vi "Raster Scan_2024-05-21+.vi"() -> ()   [LabVIEW 2024]
doc: "Shows how to move a motor to an absolute position."
uses:
  C:/Users/Behna/OneDrive/Desktop/Kinesis - Move Absolute- my work-with laser - Copy Folder/Thorlabs.MotionControl.Controls.dll
  Thorlabs.MotionControl.Controls.dll
  C:/Users/Behna/OneDrive/Desktop/Kinesis - Move Absolute- my work-with laser - Copy Folder/ThorLabs.MotionControl.KCube.DCServoCLI.dll
  ThorLabs.MotionControl.KCube.DCServoCLI.dll
  <vilib>/httpClient/LabVIEWHTTPClient.lvlib
panel:
  out "x .and. y?":bool
  in  "String":string
  out "Response":string
  in  "VISA resource name":refnum<visa-resource-name>="COM4"
  out "headers 2":string
  out "body 2":string
  out "laser run":i32
  out "remaining pulse":i32
  out "x*y":dbl
  out "GetMoveAbsolutePositionZ":dbl=6.0
  out "Numeric 2":i32
  out "Numeric":i32
  out "GetMoveAbsolutePositionX":dbl=6.0
  out "x = y?":bool
  in  "initial value_X":dbl=5.0
  in  "initial value_Z":dbl=4.0
  in  "Pulse number":string="200"
  out "body":string="{\"message\":\"success\"}"
  out "headers":string="HTTP/1.1 200 OK\r\nTransfer-Encoding: chunked\r\n\r\n"
  in  "Z-Step size":dbl=1.0
  in  "# Z-points":i32=2
  out "Z-Step":dbl[](array[numeric])=[1.0, 2.0, 3.0, 4.0, 5.0, 6.0]
  out "X-Step":dbl[](array[numeric])=[1.0, 2.0, 3.0, 4.0, 5.0, 6.0]
  in  "# X-points":i32=2
  in  "X-Step size":dbl=1.0
  in  "KCubeDCServoControl 2":refnum<k24>(container)
  in  "SerialNumber 2":string="27261646"
  in  "SerialNumber":string="27261828"
  in  "KCubeDCServoControl":refnum<k24>(container)
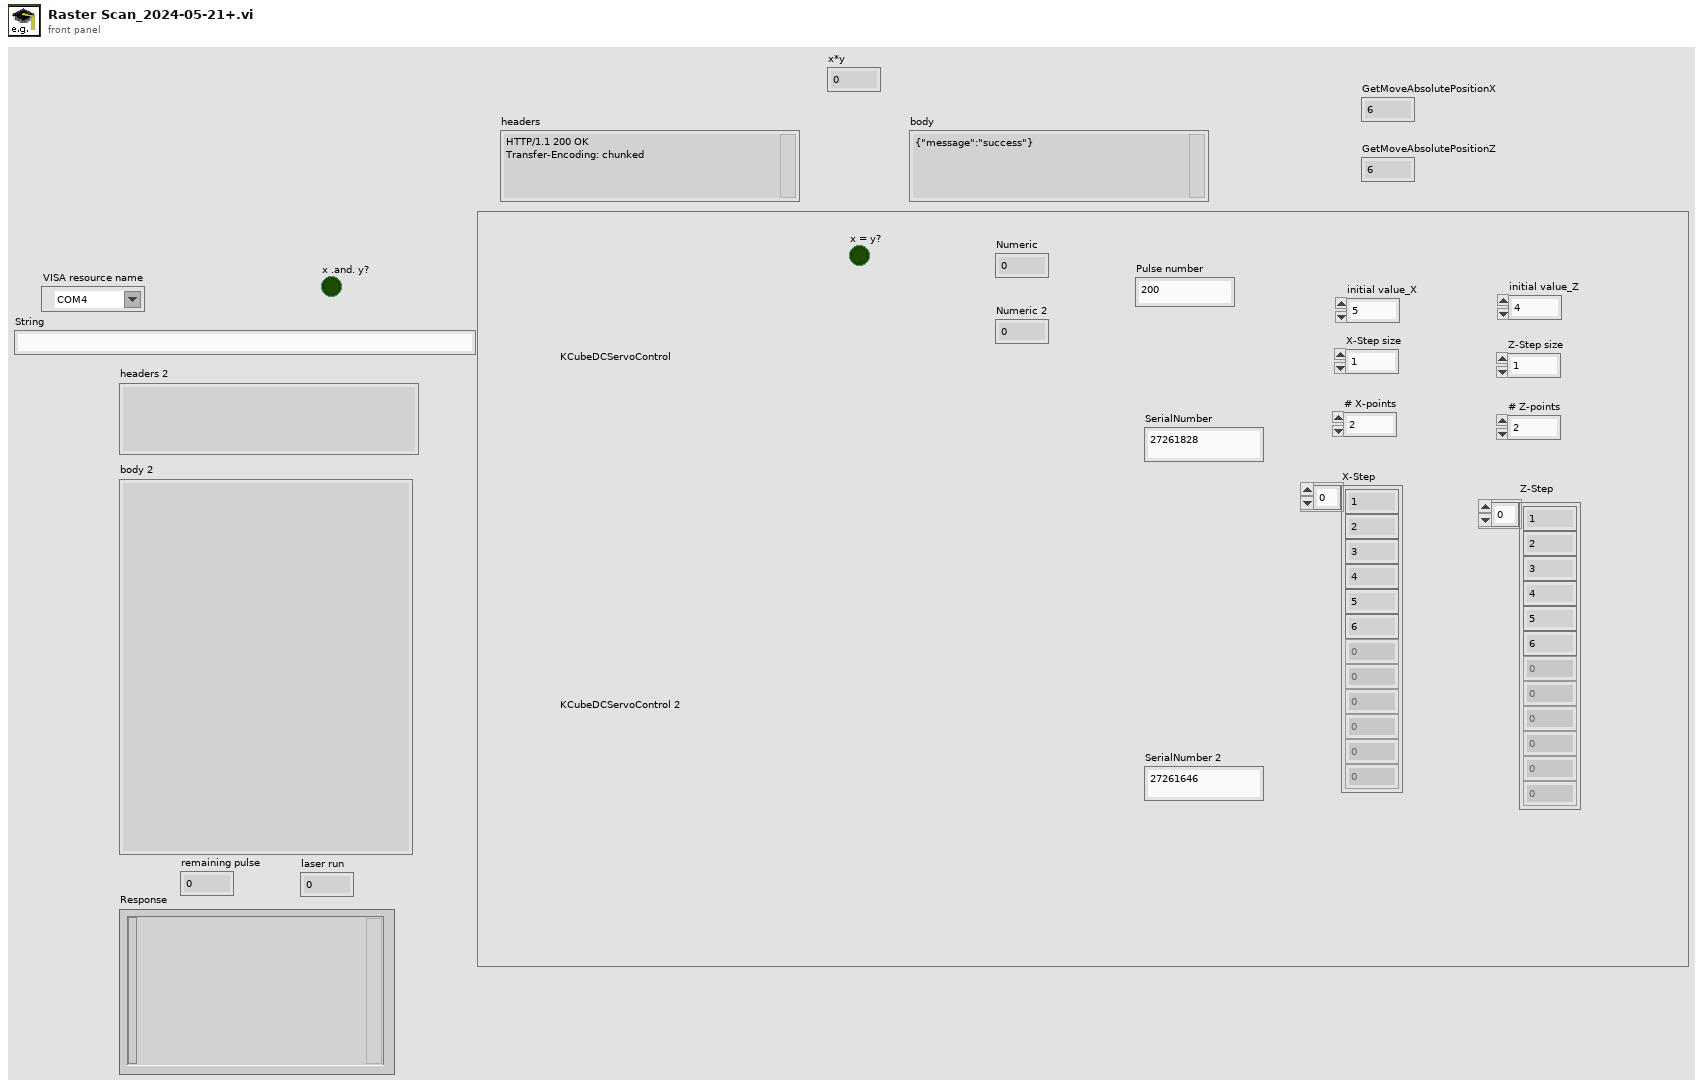
[diagram p1: front panel]
types:
  T1 = typedef "LabVIEWHTTPClient.lvlib/ClientHandle.ctl" = refnum<k1>
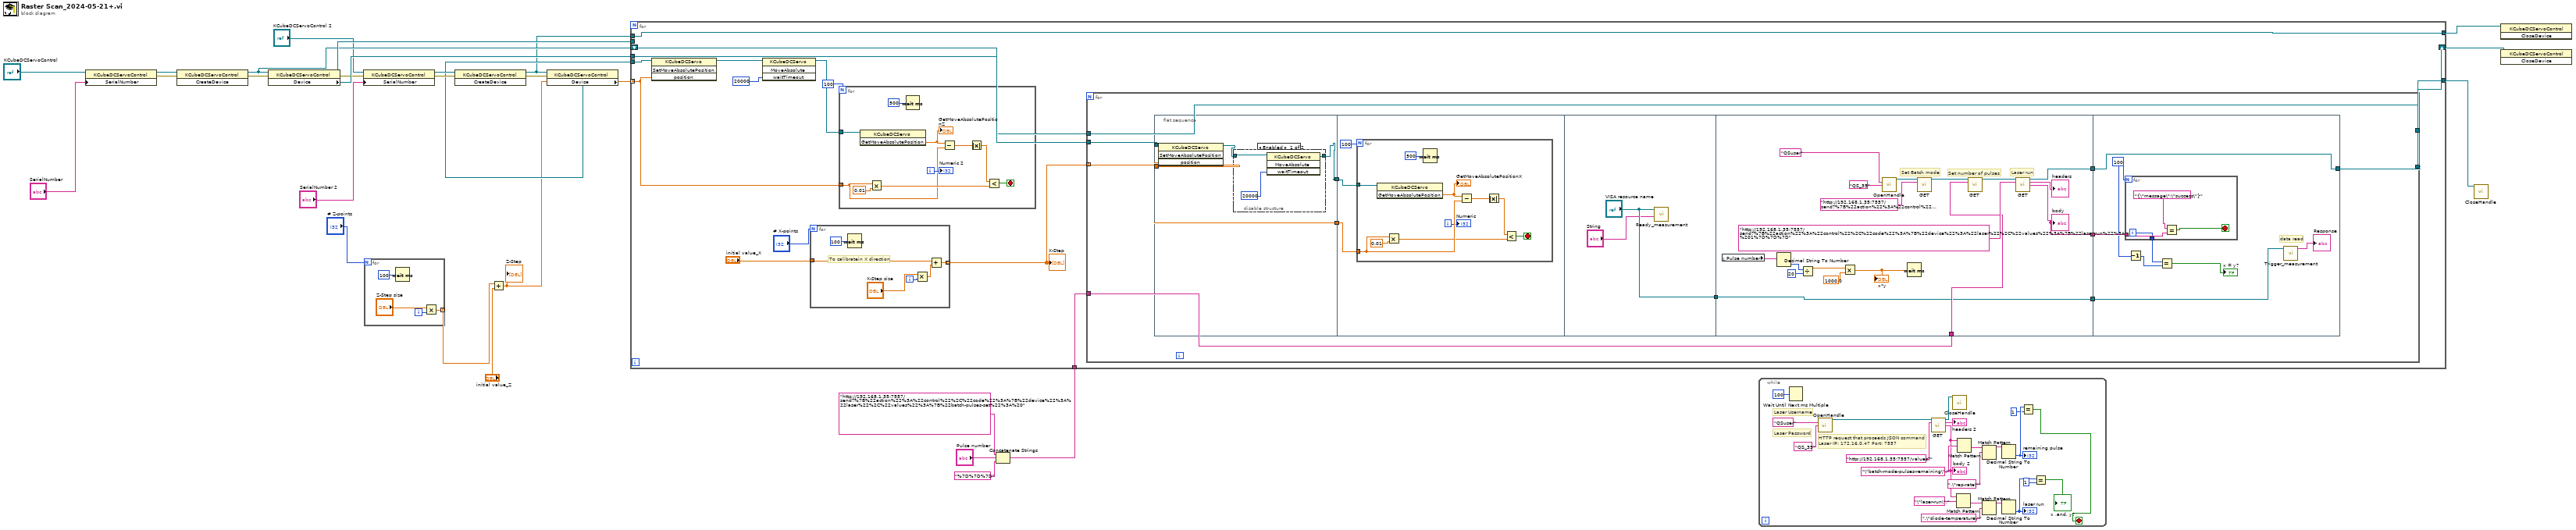
[diagram p0: block diagram]
diagram:
  n1 = property class="KCubeDCServoControl"(reference="KCubeDCServoControl", "SerialNumber"="SerialNumber") -> (reference out=w26:refnum<k24>, error out=w25:errorcluster)  [unwired: 1 in]
  n2 = invoke class="KCubeDCServoControl" method="CreateDevice"(reference=w26, error in=w25) -> (reference out=w20:refnum<k24>, error out=w24:errorcluster)  [unwired: 1 in, 1 out]
  n3 = property class="KCubeDCServoControl"(reference=w20, error in=w24) -> (reference out=w22:refnum<k24>, error out=w12:errorcluster, "Device"=w21:refnum<k24>)
  n4 = property class="KCubeDCServoControl"(reference="KCubeDCServoControl 2", error in=w12, "SerialNumber"="SerialNumber 2") -> (reference out=w15:refnum<k24>, error out=w16:errorcluster)
  n5 = for {
    N: "# Z-points" -> [_]
    tunnel: [w29] -> w3 mode=indexing
    i -> [w30]
    n6 = Wait (ms)(milliseconds to wait=u32 100) -> ()  [unwired: 1 out]
    n7 = Multiply(x="Z-Step size", y=w30) -> (x*y=w29:dbl)
  }
  n8 = invoke class="KCubeDCServoControl" method="CreateDevice"(reference=w15, error in=w16) -> (reference out=w11:refnum<k24>, error out=w17:errorcluster)  [unwired: 1 in, 1 out]
  n9 = Add(x=w3, y="initial value_Z") -> (x+y=w1:dbl[])
  "Z-Step" <- w1
  n10 = property class="KCubeDCServoControl"(reference=w11, error in=w17) -> ("Device"=w13:refnum<k24>)  [unwired: 2 out]
  n11 = Concatenate Strings("http://192.168.1.35:7557/send?%7B%22action%22%3A%22control%22%2C%22code%22%3A%7B%22device%22%3A%22laser%22%2C%22values%22%3A%7B%22batch-pulses-set%22%3A%20" ("string"), "Pulse number", "%7D%7D%7D" ("string")) -> (w4:string)
  n12 = for {
    tunnel: w22 -> [_]
    tunnel: w21 -> [w46]
    shift-right: [w44] -> w19
    shift-left: w20 -> [w45]
    tunnel: w1 -> [w33] mode=indexing
    tunnel: w13 -> [w41]
    tunnel: w11 -> [w40]
    tunnel: [w40] -> w10
    tunnel: [w38] -> w8
    tunnel: w4 -> [w36]
    n13 = invoke class="KCubeDCServo" method="SetMoveAbsolutePosition"(reference=w41, "position"=w33) -> (reference out=w43:refnum<k24>)  [unwired: 2 in, 3 out]
    n14 = invoke class="KCubeDCServo" method="MoveAbsolute"(reference=w43, "waitTimeout"=20000) -> (reference out=w34:refnum<k24>)  [unwired: 2 in, 3 out]
    n15 = for {
      N: "# X-points" -> [_]
      tunnel: [w58] -> w37 mode=indexing
      tunnel: "initial value_X" -> [w57]
      i -> [w61]
      # "To calibratein X direction"
      n16 = Wait (ms)(milliseconds to wait=u32 100) -> ()  [unwired: 1 out]
      n17 = Multiply(x="X-Step size", y=w61) -> (x*y=w59:dbl)
      n18 = Add(x=w57, y=w59) -> (x+y=w58:dbl)
    }
    "X-Step" <- w37
    n19 = for {
      N: 100 -> [_]
      tunnel: w34 -> [w55]
      tunnel: w33 -> [w47]
      i -> [w48]
      stop <- w49 stop-if-true
      n20 = invoke class="KCubeDCServo" method="GetMoveAbsolutePosition"(reference=w55) -> ("GetMoveAbsolutePosition"=w54:dbl)  [unwired: 2 in, 2 out]
      "GetMoveAbsolutePositionZ" <- w54
      n21 = Multiply(x=w47, y=0.01) -> (x*y=w50:dbl)
      n22 = Wait (ms)(milliseconds to wait=u32 500) -> ()  [unwired: 1 out]
      n23 = Subtract(x=w54, y=w47) -> (x-y=w53:dbl)
      n24 = Absolute Value(x=w53) -> (abs(x)=w51:dbl)
      n25 = Less?(x=w51, y=w50) -> (x < y?=w49:bool)
      "Numeric 2" <- w48
    }
    n26 = for {
      tunnel: w46 -> [w73]
      tunnel: w45 -> [w72]
      tunnel: [w72] -> w44
      tunnel: w37 -> [w71] mode=indexing
      tunnel: [w70] -> w38
      tunnel: w36 -> [w69]
      n27 = flat-sequence {
        tunnel: w73 -> [w77]
        tunnel: w71 -> [w74]
        tunnel: [w75] -> w68
        tunnel: [w74] -> w67
        tunnel: w67 -> [w82]
        tunnel: w68 -> [w83]
        tunnel: ["VISA resource name"] -> w63
        tunnel: [w113] -> w66
        tunnel: [w112] -> w65
        tunnel: w69 -> [w104]
        tunnel: [w96] -> w64
        tunnel: w63 -> [w96]
        tunnel: [w121] -> w70
        tunnel: w66 -> [w121]
        tunnel: w65 -> [w120]
        tunnel: w64 -> [w115]
        frame #0 {
          n28 = invoke class="KCubeDCServo" method="SetMoveAbsolutePosition"(reference=w77, "position"=w74) -> (reference out=w76:refnum<k24>)  [unwired: 2 in, 3 out]
          n29 = disable-structure shown="Enabled" {
            disable-tunnel: w76 -> [w79 _]
            disable-tunnel: [w78 _] -> w75
            frame Enabled {
              n30 = invoke class="KCubeDCServo" method="MoveAbsolute"(reference=w79, "waitTimeout"=20000) -> (reference out=w78:refnum<k24>)  [unwired: 2 in, 3 out]
            }
            frame Disabled {
            }
          }
        }
        frame #1 {
          n31 = for {
            N: 100 -> [_]
            tunnel: w83 -> [w92]
            tunnel: w82 -> [w89]
            i -> [w84]
            stop <- w85 stop-if-true
            n32 = invoke class="KCubeDCServo" method="GetMoveAbsolutePosition"(reference=w92) -> ("GetMoveAbsolutePosition"=w91:dbl)  [unwired: 2 in, 2 out]
            "GetMoveAbsolutePositionX" <- w91
            n33 = Multiply(x=w89, y=0.01) -> (x*y=w86:dbl)
            n34 = Wait (ms)(milliseconds to wait=u32 500) -> ()  [unwired: 1 out]
            n35 = Subtract(x=w91, y=w89) -> (x-y=w90:dbl)
            n36 = Absolute Value(x=w90) -> (abs(x)=w87:dbl)
            n37 = Less?(x=w87, y=w86) -> (x < y?=w85:bool)
            "Numeric" <- w84
          }
        }
        frame #2 {
          n38 = call "Ready_measurement.vi"("String"="String", "VISA resource name"="VISA resource name") -> ()  [unwired: 10 in]
        }
        frame #3 {
          # "Set Batch mode"
          # "Set number of pulses"
          # "Laser run"
          n39 = local read "Pulse number"() -> (w102:string)
          n40 = Decimal String To Number(string=w102) -> (number=w100:i32)  [unwired: 2 in, 1 out]
          n41 = Divide(x=w100, y=20) -> (x/y=w98:dbl)
          n42 = Multiply(x=w98, y=1000.0) -> (x*y=w101:dbl)
          "x*y" <- w101
          n43 = call <vilib>:"OpenHandle.vi"("username"="QSuser", "password"="QS_35") -> ("client handle out"=w97:T1)  [unwired: 12 in, 1 out]
          n44 = Wait (ms)(milliseconds to wait=w101) -> ()  [unwired: 1 out]
          n45 = call <vilib>:"GET.vi"("client handle"=w97, "url"="http://192.168.1.35:7557/send?%7B%22action%22%3A%22control%22%2C%22code%22%3A%7B%22device%22%3A%22laser%22%2C%22values%22%3A%7B%22batch-mode%22%3A %201%7D%7D%7D") -> ("client handle out"=w109:T1)  [unwired: 10 in, 3 out]
          n46 = call <vilib>:"GET.vi"("client handle"=w109, "url"=w104) -> ("client handle out"=w107:T1)  [unwired: 10 in, 3 out]
          n47 = call <vilib>:"GET.vi"("client handle"=w107, "url"="http://192.168.1.35:7557/send?%7B%22action%22%3A%22control%22%2C%22code%22%3A%7B%22device%22%3A%22laser%22%2C%22values%22%3A%7B%22laser-run%22%3A%201%7D%7D%7D") -> ("client handle out"=w113:T1, "headers"=→"headers":string, "body"=w112:string)  [unwired: 10 in, 1 out]
          "body" <- w112
        }
        frame #4 {
          w117 = 100
          # "data read"
          n48 = for {
            N: w117 -> [_]
            tunnel: w120 -> [w124]
            tunnel: [w122] -> w119
            i -> [w122]
            stop <- w123 stop-if-true
            n49 = Equal?(x="{\"message\":\"success\"}", y=w124) -> (x = y?=w123:bool)
          }
          n50 = Decrement(x=w117) -> (x-1=w118:i32)
          n51 = Equal?(x=w119, y=w118) -> (x = y?=→"x = y?":bool)
          n52 = call "Trigger_measurement.vi"("VISA resource name"=w115) -> ("Response"=→"Response":string)  [unwired: 10 in]
        }
      }
    }
  }
  n53 = while {
    stop <- w126 stop-if-true
    # "HTTP request that proceeds JSON command\nLaser IP: 172.16.0.47 Port: 7557"
    # "Laser Password"
    # "Laser Username"
    n54 = Wait Until Next ms Multiple(millisecond multiple=u32 100) -> ()  [unwired: 1 out]
    n55 = call <vilib>:"OpenHandle.vi"("username"="QSuser", "password"="QS_35") -> ("client handle out"=w146:T1)  [unwired: 12 in, 1 out]
    n56 = call <vilib>:"GET.vi"("client handle"=w146, "url"="http://192.168.1.35:7557/values?") -> ("client handle out"=w143:T1, "headers"=→"headers 2":string, "body"=w132:string)  [unwired: 10 in, 1 out]
    "body 2" <- w132
    n57 = call <vilib>:"CloseHandle.vi"("client handle"=w143) -> ()  [unwired: 14 in, 1 out]
    n58 = Match Pattern(string=w132, regular expression="\"laser-run\":") -> (after substring=w138:string)  [unwired: 1 in, 3 out]
    n59 = Match Pattern(string=w132, regular expression="\"batch-mode-pulses-remaining\":") -> (after substring=w135:string)  [unwired: 1 in, 3 out]
    n60 = Match Pattern(string=w135, regular expression=",\"rep-rate\"") -> (before substring=w133:string)  [unwired: 1 in, 3 out]
    n61 = Match Pattern(string=w138, regular expression=",\"diode-temperature\"") -> (before substring=w137:string)  [unwired: 1 in, 3 out]
    n62 = Decimal String To Number(string=w133) -> (number=w129:i32)  [unwired: 2 in, 1 out]
    "remaining pulse" <- w129
    n63 = Decimal String To Number(string=w137) -> (number=w131:i32)  [unwired: 2 in, 1 out]
    "laser run" <- w131
    n64 = Equal?(x=w129, y=1) -> (x = y?=w126:bool)
    n65 = Equal?(x=w131, y=1) -> (x = y?=→"x .and. y?":bool)
  }
  n66 = call <vilib>:"CloseHandle.vi"("client handle"=w8) -> ()  [unwired: 14 in, 1 out]
  n67 = invoke class="KCubeDCServoControl" method="CloseDevice"(reference=w10) -> ()  [unwired: 2 in, 3 out]
  n68 = invoke class="KCubeDCServoControl" method="CloseDevice"(reference=w19) -> ()  [unwired: 2 in, 3 out]
